vi "DiscArchiver.empty file name.vi"() -> (16 "emptyString":string)   [LabVIEW 2014, in "DiscArchiver.lvlib"]
doc: "Returns an empty string for the data file name. The string has a fixed length and is filled with \"\\0\" characters."
uses:
  DiscArchiver.lvlib
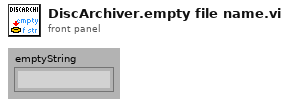
[diagram p1: front panel]
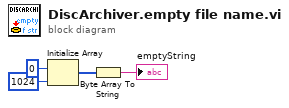
[diagram p0: block diagram]
diagram:
  n1 = Initialize Array(u8 0, 1024 ("dimension size")) -> (w2:u8[])
  n2 = Byte Array To String(unsigned byte array=w2) -> (string=→"emptyString":string)
